vi "Write Waveform.vi"(8 "error in (no error)":errorcluster, 10 "I-V parameters":T1={"Start magnitude"=2e-05, "Magnitude increment"=5e-05, "Number of pulses"=50, "Baseline length"=0, "Ramp length"=0, "Top  length"=0, "Threshold "=2e-06, "Processing Delay"=0, "Valhalla range"=0.001, "Interpolation"=64} {"Valhalla range" format="%#_6pA"; "Processing Delay" format="%dpts"; "Threshold" format="%#_6pV"; "Top  length" format="%dpts"; "Ramp length" format="%dpts"; "Baseline length" format="%dpts"; "Magnitude increment" format="%#_6pA"; "Start magnitude" format="%#_6pA"}, 11 "RP Instrument in":refnum<class "RP Instrument.lvclass">) -> (0 "error out":errorcluster, 2 "Output Waveform":i16[](graph), 3 "RP Instrument out":refnum<class "RP Instrument.lvclass">)   [LabVIEW 2016, in "RP Instrument.lvclass"]
uses:
  RP Instrument.lvclass
  Waform generation/I-V parameters.ctl
  RP Instrument.lvclass/RP Instrument.ctl
  RP Communicator/RP Communicator.lvclass
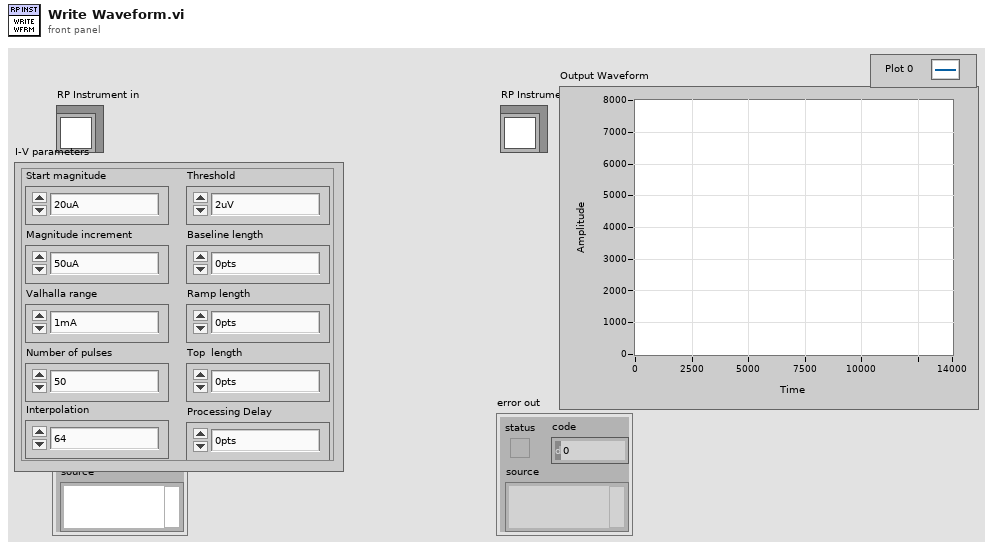
[diagram p1: front panel]
types:
  T1 = typedef "I-V parameters.ctl" = cluster{"Start magnitude":dbl, "Magnitude increment":dbl, "Number of pulses":i32, "Baseline length":i32, "Ramp length":i32, "Top  length":i32, "Threshold ":dbl, "Processing Delay":u16, "Valhalla range":dbl, "Interpolation":i32}
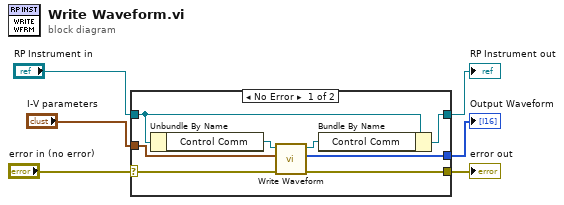
[diagram p0: block diagram]
diagram:
  n1 = case shown="No Error" "error in (no error)" {
    selector: "error in (no error)" -> [w9 w16]
    tunnel: [w8 w16] -> w5
    tunnel: [w12 w15] -> w3
    tunnel: "RP Instrument in" -> [w14 w15]
    tunnel: "I-V parameters" -> [w10 _]
    tunnel: [w7 _] -> w1
    frame No Error {
      n2 = Unbundle By Name(w14) -> ("Control Comm"=w13:refnum<class "RP Communicator.lvclass">)
      n3 = call-dynamic "Write Waveform.vi"("error in (no error)"=w9, "I-V parameters"=w10, "RP Communicator in"=w13) -> ("error out"=w8:errorcluster, "Output Waveform"=w7:i16[], "RP Communicator out"=w11:refnum<class "RP Communicator.lvclass">)  [unwired: 6 in]
      n4 = Bundle By Name(cluster=w14, "Control Comm"=w11) -> (w12:refnum<class "RP Instrument.lvclass">)
    }
    frame Error {
    }
  }
  "error out" <- w5
  "RP Instrument out" <- w3
  "Output Waveform" <- w1
